vi "SwapInstanceVIUnusedName2 58.vi"(6 "Bindata & descr in":T1, 7 "type":sgl, 8 "error in (no error)":errorcluster, 9 "dims":u8=3 min=1 max=3, 11 "kwarg_name":string="testarg") -> (0 "error out":errorcluster, 1 "Array 3D":sgl[][][](array[numeric]) format="%.2f", 2 "Array 2D":sgl[][](array[numeric]) format="%.2f", 3 "Array 1D":sgl[](array[numeric]) format="%.2f", 4 "Bindata & descr out":T1, 5 "bindata":u8[](array[numeric]))   [LabVIEW 2018]
uses:
  Bindata&description.ctl
  Bindata description.ctl
  1a5d6881-bca9-4a1b-b0ee-b1572d0d71c2.vi
  c4985320-b457-44c4-bbda-591843926ead.vi
  538973bc-dc26-4b4c-a705-cbe7740b2b08.vi
  d1ffc927-7398-4d90-9cb0-4b6e9eb9afd5.vi
  c4985320-b457-44c4-bbda-591843926ead.vi/0e9a7685-389e-46ee-b9ae-44a36e2b7ad8.vi
  538973bc-dc26-4b4c-a705-cbe7740b2b08.vi/21411a45-59e3-4942-9a2b-5773b08ed5b9.vi
  d1ffc927-7398-4d90-9cb0-4b6e9eb9afd5.vi/e00ddee1-3fb3-4725-8aa9-a19eaaaf1f80.vi
  c4985320-b457-44c4-bbda-591843926ead.vi/0e9a7685-389e-46ee-b9ae-44a36e2b7ad8.vi/96658f3e-b8f5-401a-a6fb-5cdaa814c42e.vi
  538973bc-dc26-4b4c-a705-cbe7740b2b08.vi/21411a45-59e3-4942-9a2b-5773b08ed5b9.vi/65a4f665-78c0-4ecb-9edc-d2675a269e53.vi
  d1ffc927-7398-4d90-9cb0-4b6e9eb9afd5.vi/e00ddee1-3fb3-4725-8aa9-a19eaaaf1f80.vi/63b03a6a-42a0-4ff6-9395-398ede17ba95.vi
  c4985320-b457-44c4-bbda-591843926ead.vi/0e9a7685-389e-46ee-b9ae-44a36e2b7ad8.vi/96658f3e-b8f5-401a-a6fb-5cdaa814c42e.vi/29a54583-2bd5-4a38-a614-c4701d3c2139.vi
  538973bc-dc26-4b4c-a705-cbe7740b2b08.vi/21411a45-59e3-4942-9a2b-5773b08ed5b9.vi/65a4f665-78c0-4ecb-9edc-d2675a269e53.vi/f7253fb2-adb9-4d5a-819c-638c3c29e0b4.vi
  d1ffc927-7398-4d90-9cb0-4b6e9eb9afd5.vi/e00ddee1-3fb3-4725-8aa9-a19eaaaf1f80.vi/63b03a6a-42a0-4ff6-9395-398ede17ba95.vi/e7bdb3d7-3cf8-4b9d-b515-e3fbd54a74d4.vi
  check ID validity.vi
  LV-Julia_ZMQ-Roundtrip_lib.lvlib
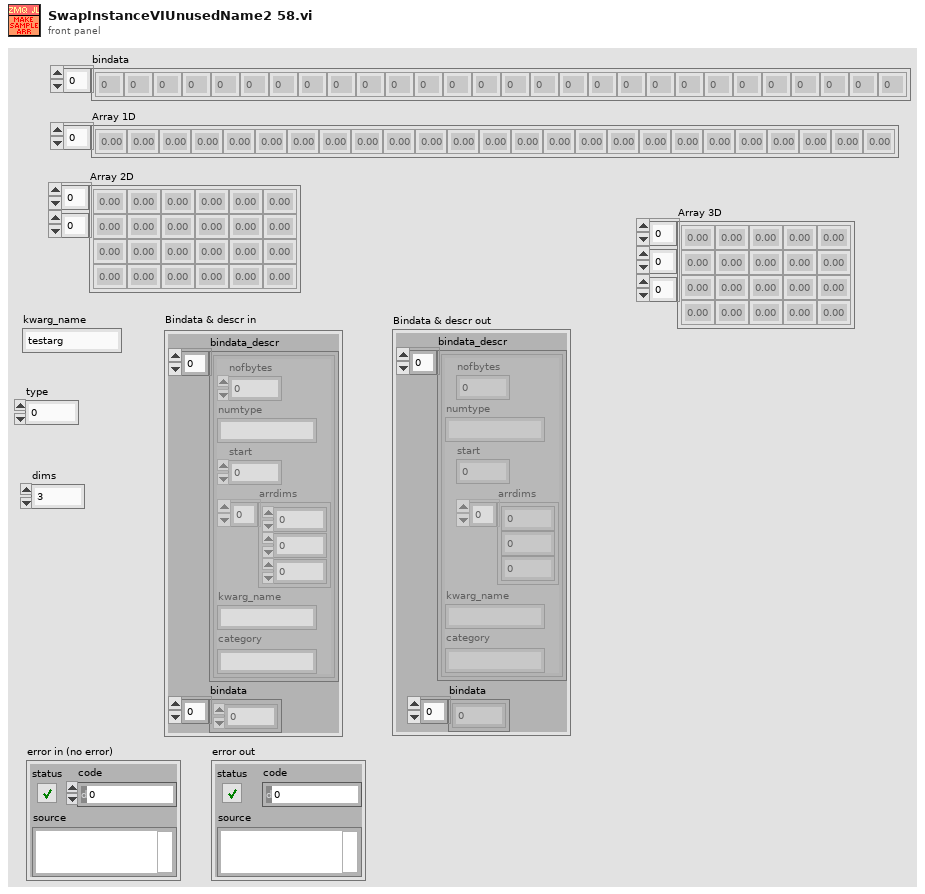
[diagram p1: front panel]
types:
  T1 = typedef "Bindata&description.ctl" = cluster{"bindata_descr":T2[], "bindata":u8[]}
  T2 = typedef "LV-Julia_ZMQ-Roundtrip_lib.lvlib/Bindata description.ctl" = cluster{"nofbytes":i32, "numtype":string, "start":i32, "arrdims":i32[], "kwarg_name":string, "category":string}
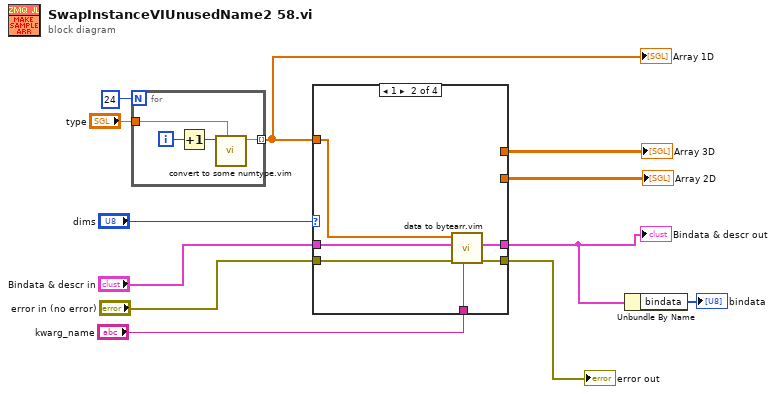
[diagram p0: block diagram]
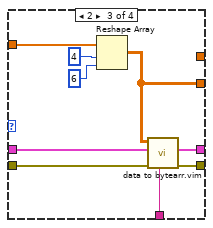
[diagram p3: hidden frame]
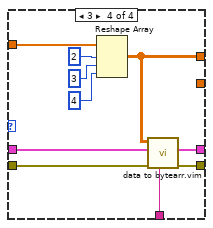
[diagram p4: hidden frame]
diagram:
  n1 = for {
    N: 24 -> [_]
    tunnel: [w14] -> w11 mode=indexing
    tunnel: "type" -> [w13]
    i -> [w16]
    n2 = Increment(x=w16) -> (x+1=w15:i32)
    n3 = call "convert to some numtype.vim"("type"=w13, "Numeric in"=w15) -> ("Numeric out"=w14:sgl)  [unwired: 9 in]
  }
  "Array 1D" <- w11
  n4 = case shown="1" "dims" {
    tunnel: [_ _ _ w42] -> w12
    tunnel: w11 -> [_ w23 w30 w38]
    tunnel: "kwarg_name" -> [_ w22 w29 w37]
    tunnel: "error in (no error)" -> [w17 w21 w28 w36]
    tunnel: [w17 w20 w27 w35] -> w5
    tunnel: [_ w19 w26 w34] -> w2
    tunnel: [_ _ w25 _] -> w4
    tunnel: "Bindata & descr in" -> [_ w18 w24 w33]
    frame 0, Default {
    }
    frame 1 {
      n5 = call "data to bytearr.vim"("kwarg_name"=w22, "error in (no error)"=w21, "Bindata & descr in"=w18, "data in"=w23) -> ("error out"=w20:errorcluster, "Bindata & descr out"=w19:T1)  [unwired: 5 in, 1 out]
    }
    frame 2 {
      n6 = Reshape Array(w30, 4 ("dimension size"), 6 ("dimension size")) -> (w25:sgl[][])
      n7 = call "data to bytearr.vim"("kwarg_name"=w29, "error in (no error)"=w28, "Bindata & descr in"=w24, "data in"=w25) -> ("error out"=w27:errorcluster, "Bindata & descr out"=w26:T1)  [unwired: 5 in, 1 out]
    }
    frame 3 {
      n8 = Reshape Array(w38, 2 ("dimension size"), 3 ("dimension size"), 4 ("dimension size")) -> (w42:sgl[][][])
      n9 = call "data to bytearr.vim"("kwarg_name"=w37, "error in (no error)"=w36, "Bindata & descr in"=w33, "data in"=w42) -> ("error out"=w35:errorcluster, "Bindata & descr out"=w34:T1)  [unwired: 5 in, 1 out]
    }
  }
  "Array 3D" <- w12
  "Bindata & descr out" <- w2
  "error out" <- w5
  "Array 2D" <- w4
  n10 = Unbundle By Name(w2) -> ("bindata"=→"bindata":u8[])
